vi "Update Class with Parent.vi"(8 "error in (no error)":errorcluster, 11 "QControl Creation in":refnum<class "QControl Creation.lvclass">) -> (0 "error out":errorcluster, 3 "QControl Creation (dup)":refnum<class "QControl Creation.lvclass">)   [LabVIEW 2015, in "QControl Creation.lvclass"]
doc: "<b> </b> <b> </b>\n©2016 Q Software Innovations, LLC (QSI)\nwritten by Quentin Alldredge\nproduced in LabVIEW 2015\n\nsupport@qsoftwareinnovations.com\nwww.qsoftwareinnovations.com\n\nAll rights reserved.\n\nRedistribution and use in source and binary forms, with or without modification, are permitted provided that the following conditions are met:\n\n * Redistributions of source code must retain the above copyright notice, this list of conditions and the following disclaimer.\n * Redistributions in binary form must reproduce the above copyright notice, this list of conditions and the following disclaimer in the documentation and/or other materials provided with the distribution.\n * Neither the name of Q Software Innovations, LLC. nor the names of its contributors may be used to endorse or promote products derived from this software without specific prior written permission.\n\nTHIS SOFTWARE IS PROVIDED BY THE COPYRIGHT HOLDERS AND CONTRIBUTORS \"AS IS\" AND ANY EXPRESS OR IMPLIED WARRANTIES, INCLUDING, BUT NOT LIMITED TO, THE IMPLIED WARRANTIES OF MERCHANTABILITY AND FITNESS FOR A PARTICULAR PURPOSE ARE DISCLAIMED. IN NO EVENT SHALL THE COPYRIGHT OWNER OR CONTRIBUTORS BE LIABLE FOR ANY DIRECT, INDIRECT, INCIDENTAL, SPECIAL, EXEMPLARY, OR CONSEQUENTIAL DAMAGES (INCLUDING, BUT NOT LIMITED TO, PROCUREMENT OF SUBSTITUTE GOODS OR SERVICES; LOSS OF USE, DATA, OR PROFITS; OR BUSINESS INTERRUPTION) HOWEVER CAUSED AND ON ANY THEORY OF LIABILITY, WHETHER IN CONTRACT, STRICT LIABILITY, OR TORT (INCLUDING NEGLIGENCE OR OTHERWISE) ARISING IN ANY WAY OUT OF THE USE OF THIS SOFTWARE, EVEN IF ADVISED OF THE POSSIBILITY OF SUCH DAMAGE."
uses:
  QControl Creation.lvclass
  QControl Creation.lvclass/QControl Creation.ctl
  <vilib>/Utility/error.llb/Error Cluster From Error Code.vi
  <vilib>/ErrorRing/Error Ring.xnode
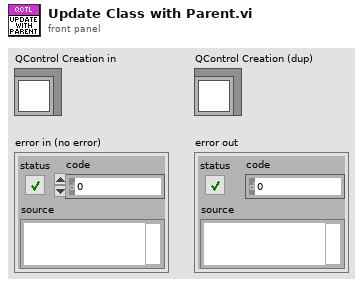
[diagram p1: front panel]
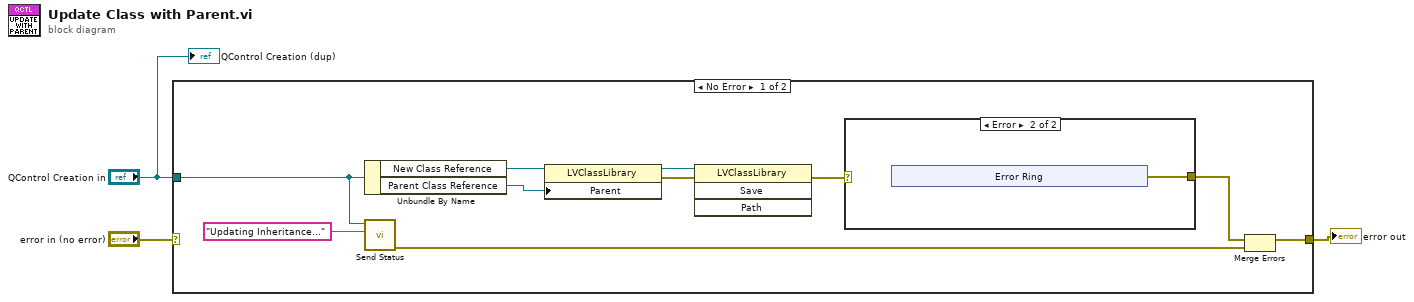
[diagram p0: block diagram]
diagram:
  n1 = case shown="No Error" "error in (no error)" {
    selector: "error in (no error)" -> [_ w21]
    tunnel: [w7 w21] -> w2
    tunnel: "QControl Creation in" -> [w8 _]
    frame No Error {
      n2 = Unbundle By Name(w8) -> ("New Class Reference"=w13:refnum<vi>, "Parent Class Reference"=w10:refnum<vi>)
      n3 = call "Send Status.vi"("Status"="Updating Inheritance..." ("Value"), "QControl Creation in"=w8) -> ("error out (dup)"=w6:errorcluster)  [unwired: 8 in, 1 out]
      n4 = property class="LVClassLibrary"(reference=w13, "Parent"=w10) -> (reference out=w11:refnum<vi>, error out=w12:errorcluster)  [unwired: 1 in]
      n5 = invoke class="LVClassLibrary" method="Save"(reference=w11, error in=w12) -> (error out=w5:errorcluster)  [unwired: 2 in, 3 out]
      n6 = case shown="Error" w5 {
        selector: w5 -> [w14 _]
        tunnel: [w14 w15] -> w4
        frame No Error {
        }
        frame Error {
          n7 = xnode "Error Ring"() -> ("error out"=w15:errorcluster)
        }
      }
      n8 = Merge Errors(w4, w6) -> (w7:errorcluster)
    }
    frame Error {
    }
  }
  "error out" <- w2
  "QControl Creation (dup)" <- "QControl Creation in"
